vi "writeLimitsFirgelli.vi"(6 "select":enum16{"Retract", "Extend"}(ring), 8 "error in (no error)":errorcluster, 9 "maxLength":dbl format="%.2f", 10 "limit":dbl format="%.2f", 11 "handleIn":u32 format="%x") -> (0 "error out":errorcluster, 1 "regSetting":u16, 2 "pDataOut":u8[](array[numeric]), 3 "handleOut":u32 format="%x")   [LabVIEW 2016]
doc: "0x02 SET_RETRACT_LIMIT and 0x03 SET_EXTEND_LIMIT\nThese are the values that are set with the Limits Potentiometers. Setting the\nExtend_Limit to 1023 and the Retract_Limit to zero will allow movement over the full range. However, it is recommended to offset these values to ensure the actuator is never driven into the physical end stops. This increases cycle life considerably. To set the desired limits take the distance (mm) from the physical stop you wish to limit the actuator to, and plug it into the following equation.\n\nWritten by: Complete Automated Solutions\nwww.CompleteAutomatedSolutions.com"
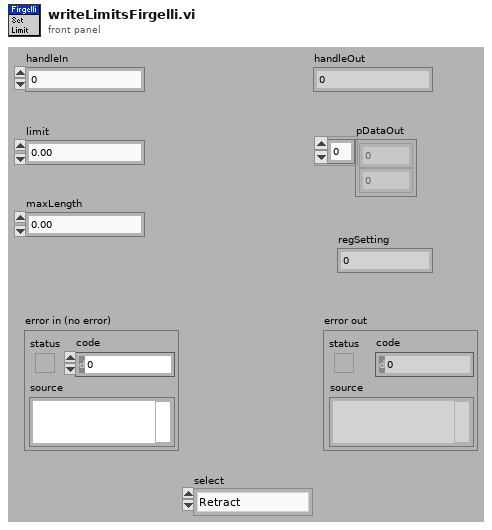
[diagram p1: front panel]
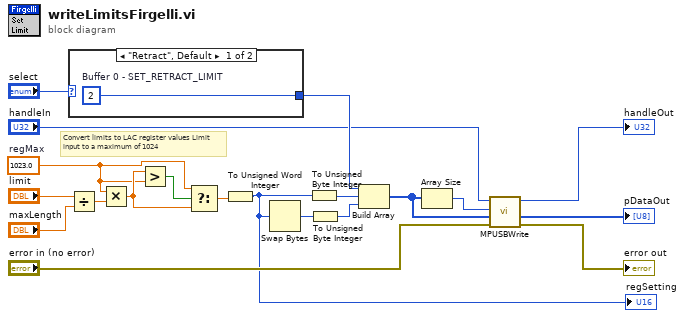
[diagram p0: block diagram]
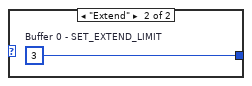
[diagram p2: hidden frame]
diagram:
  w2 = 1023.0  # regMax
  # "Convert limits to LAC register values Limit\ninput to a maximum of 1024"
  n1 = case shown="\"Retract\", Default" "select" {
    tunnel: [w21 w22] -> w17
    frame "Retract", Default {
      w21 = u8 2  # Buffer 0 - SET_RETRACT_LIMIT
    }
    frame "Extend" {
      w22 = u8 3  # Buffer 0 - SET_EXTEND_LIMIT
    }
  }
  n2 = Divide(x="limit", y="maxLength") -> (x/y=w10:dbl)
  n3 = Multiply(x=w2, y=w10) -> (x*y=w3:dbl)
  n4 = Greater?(x=w3, y=w2) -> (0:w4:bool)
  n5 = Select(t=w2, s=w4, f=w3) -> (s? t:f=w5:dbl)
  n6 = To Unsigned Word Integer(number=w5) -> (unsigned 16bit integer=w9:u16)
  "regSetting" <- w9
  n7 = Swap Bytes(anything=w9) -> (byte swapped=w20:u16)
  n8 = To Unsigned Byte Integer(number=w9) -> (unsigned 8bit integer=w18:u8)
  n9 = To Unsigned Byte Integer(number=w20) -> (unsigned 8bit integer=w19:u8)
  n10 = Build Array(w17, w18, w19) -> (w15:u8[])
  n11 = Array Size(array=w15) -> (size(s)=w16:i32)
  n12 = call "MPUSBWrite.vi"("error in (no error)"="error in (no error)", "pDataIn"=w15, "dwLen"=w16, "handleIn"="handleIn") -> ("error out"=→"error out":errorcluster, "pDataOut"=→"pDataOut":u8[], "handleOut"=→"handleOut":u32)  [unwired: 2 in, 3 out]
